vi "Build Message with Arguments(Auto Check).vi"(5 "State with Arguments":string, 7 "Arguments (\"\")":string, 9 "Target Module (\"\")":string) -> (6 "State with Arguments out":string)   [LabVIEW 2020, in "Communicable State Machine.lvlib"]
doc: "Builds a message that contains arguments for CSM. This VI will parse \"State with Arguments\" for message type, message string, arguments and target module from input <b>State with Arguments</b> and replace corresponding parts in the message with input values. The message type from input <b>State with Arguments</b> will be used.\n\n<B>For Example:</B>\n\nIf <b>State with Arguments</b> input is \"API: DoSth\"\n<b>Arguments (\"\")</b> input is \"Arguments\"\n<b>Target Module (\"\")</b> input is \"Callee\"\nThen result string is \"API: DoSth >> Arguments\" as no message symbol is detected.\n\nIf <b>State with Arguments</b> input is \"API: DoSth >> Arguments -> Callee\"\n<b>Arguments (\"\")</b> input is \"NewArguments\"\n<b>Target Module (\"\")</b> input is \"\"\nThen result string is \"API: DoSth >> NewArguments -> Callee\"\n\nIf <b>State with Arguments</b> input is \"API: DoSth >> Arguments -> Callee\"\n<b>Arguments (\"\")</b> input is \"NewArguments\"\n<b>Target Module (\"\")</b> input is \"NewCallee\"\nThen result string is \"API: DoSth >> NewArguments -> NewCallee\"\n\nIf <b>State with Arguments</b> input is \"API: DoSth >> Arguments -> Callee\"\n<b>Arguments (\"\")</b> input is \"\"\n<b>Target Module (\"\")</b> input is \"NewCallee\"\nThen result string is \"API: DoSth -> NewCallee\"\n\nIf <b>State with Arguments</b> input is \"API: DoSth >> Arguments -@ Callee\"\n<b>Arguments (\"\")</b> input is \"NewArguments\"\n<b>Target Module (\"\")</b> input is \"\"\nThen result string is \"API: DoSth >> NewArguments -@ Callee\"\n\n<b>Inputs:</b>\n - <b>State with Arguments</b>: Input Message which might contain Arguments or target Module\n - <b>Arguments (\"\")</b>: The arguments which will be used to replace arguments in <b>State with Arguments</b>. if empty, no arguments will be included in output strings.\n - <b>Target Module (\"\")</b>: The target which will be used to replace target in <b>State with Arguments</b>. if empty, target in <b>State with Arguments</b> will be used.\n\n<b>Outputs:</b>\n - <b>State with Arguments</b>: String stands for state with arguments"
uses:
  Communicable State Machine.lvlib
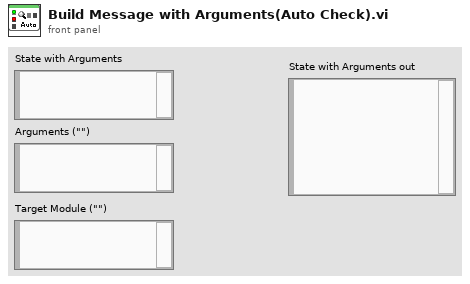
[diagram p1: front panel]
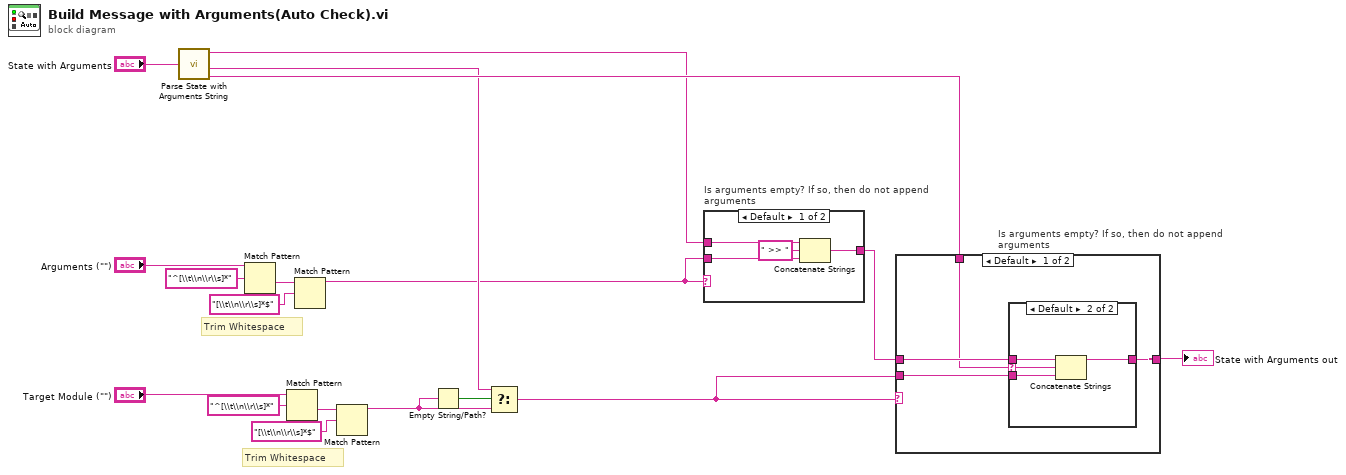
[diagram p0: block diagram]
diagram:
  # "Trim Whitespace"
  # "Trim Whitespace"
  n1 = call "Parse State with Arguments String.vi"("State with Arguments"="State with Arguments") -> ("State"=w2:string, "Target Module"=w6:string, "Message Symbol"=w8:string)  [unwired: 6 in, 1 out]
  n2 = Match Pattern(string="Arguments (\"\")", regular expression="^[\\t\\n\\r\\s]*") -> (after substring=w17:string)  [unwired: 1 in, 3 out]
  n3 = Match Pattern(string="Target Module (\"\")", regular expression="^[\\t\\n\\r\\s]*") -> (after substring=w13:string)  [unwired: 1 in, 3 out]
  n4 = Match Pattern(string=w17, regular expression="[\\t\\n\\r\\s]*$") -> (before substring=w1:string)  [unwired: 1 in, 3 out]
  n5 = Match Pattern(string=w13, regular expression="[\\t\\n\\r\\s]*$") -> (before substring=w4:string)  [unwired: 1 in, 3 out]
  n6 = Empty String/Path?(string/path=w4) -> (empty?=w7:bool)
  n7 = Select(t=w6, s=w7, f=w4) -> (s? t:f=w3:string)
  n8 = case "Is arguments empty? If so, then do not append arguments" shown="Default" w1 {
    tunnel: [w19 w23] -> w10
    tunnel: w2 -> [w22 w23]
    tunnel: w1 -> [w20 _]
    frame Default {
      n9 = Concatenate Strings(w22, " >> " ("string"), w20) -> (w19:string)
    }
    frame "" {
    }
  }
  n10 = case "Is arguments empty? If so, then do not append arguments" shown="Default" w3 {
    tunnel: [w25 w33] -> w11
    tunnel: w10 -> [w27 w33]
    tunnel: w3 -> [w26 _]
    tunnel: w8 -> [w24 _]
    frame Default {
      n11 = case shown="Default" w24 {
        selector: w24 -> [_ w29]
        tunnel: w27 -> [w28 w32]
        tunnel: w26 -> [_ w31]
        tunnel: [w28 w30] -> w25
        frame "" {
        }
        frame Default {
          n12 = Concatenate Strings(w32, w29, w31) -> (w30:string)
        }
      }
    }
    frame "" {
    }
  }
  "State with Arguments out" <- w11
